vi "Compile Knock Sensor 1.0 Data.vi"(7 "RIO Address":string, 8 "error in (no error)":errorcluster, 11 "Device Item Ref in":T3 format="%.0x") -> (0 "error out":errorcluster, 2 "Knock Sensors":T1[](array[typedef]), 3 "Device Item Ref out":T3 format="%.0x")   [LabVIEW 2020, in "Engine Simulation Toolkit System Explorer.lvlib"]
uses:
  Engine Simulation Toolkit System Explorer.lvlib
  <vilib>/NI VeriStand/Custom Device API/Custom Device Item Ref.ctl
  Shared/1.0 Knock Sensor Engine Data.ctl
  Shared/1.0 Knock Sensor FIFO Idxs.ctl
  Knock Low Freq Setting.ctl
  Shared/Constants and GUIDs.vi
  <vilib>/NI VeriStand/Custom Device Tools/Custom Device Utility Library/NI VeriStand - Search for Item by GUID.vi
  Shared/Properties.vi
  <vilib>/NI VeriStand/Custom Device API/Get Item Property (String).vi
  <vilib>/NI VeriStand/Custom Device API/Get Item Property (U16).vi
  <vilib>/NI VeriStand/Custom Device API/Get Item Property (Double).vi
  Shared/Engine Simulation Toolkit Shared.lvlib
  <vilib>/NI VeriStand/Custom Device Tools/Custom Device Utility Library/Custom Device Utility Library.lvlib
  <vilib>/NI VeriStand/Custom Device API/Custom Device API.lvlib
  <vilib>/rvi/Analysis/host/Public/NI_FpgaMspHost.lvlib
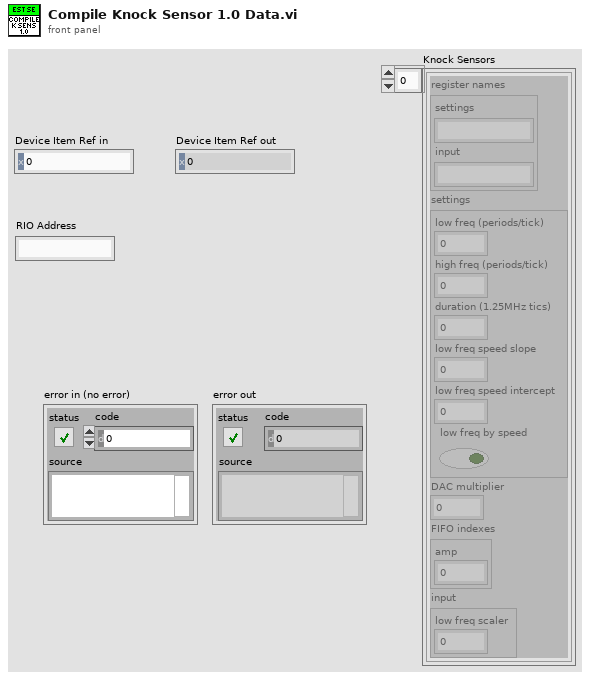
[diagram p1: front panel]
types:
  T1 = typedef "Engine Simulation Toolkit Shared.lvlib/1.0 Knock Sensor Engine Data.ctl" = cluster{"register names":cluster{"settings":string, "input":string}, "settings":cluster{"low freq (periods/tick)":fxp<+,32,0>, "high freq (periods/tick)":fxp<+,32,0>, "duration (1.25MHz tics)":fxp<+,18,18>, "low freq speed slope":fxp<+,16,-3>, "low freq speed intercept":fxp<+,10,-10>, "low freq by speed":bool}, "DAC multiplier":dbl, "FIFO indexes":T2, "input":cluster{"low freq scaler":fxp<+,10,0>}}
  T2 = typedef "Engine Simulation Toolkit Shared.lvlib/1.0 Knock Sensor FIFO Idxs.ctl" = cluster{"amp":i32}
  T3 = typedef "Custom Device API.lvlib/Custom Device Item Ref.ctl" = u64
  T4 = typedef "Engine Simulation Toolkit Shared.lvlib/Channel.ctl" = cluster{"Name":string, "Units":string, "Default":dbl, "Description":string, "Scalable":bool}
  T5 = typedef "Engine Simulation Toolkit System Explorer.lvlib/Knock Low Freq Setting.ctl" = enum16{"Manually", "As function of speed"}
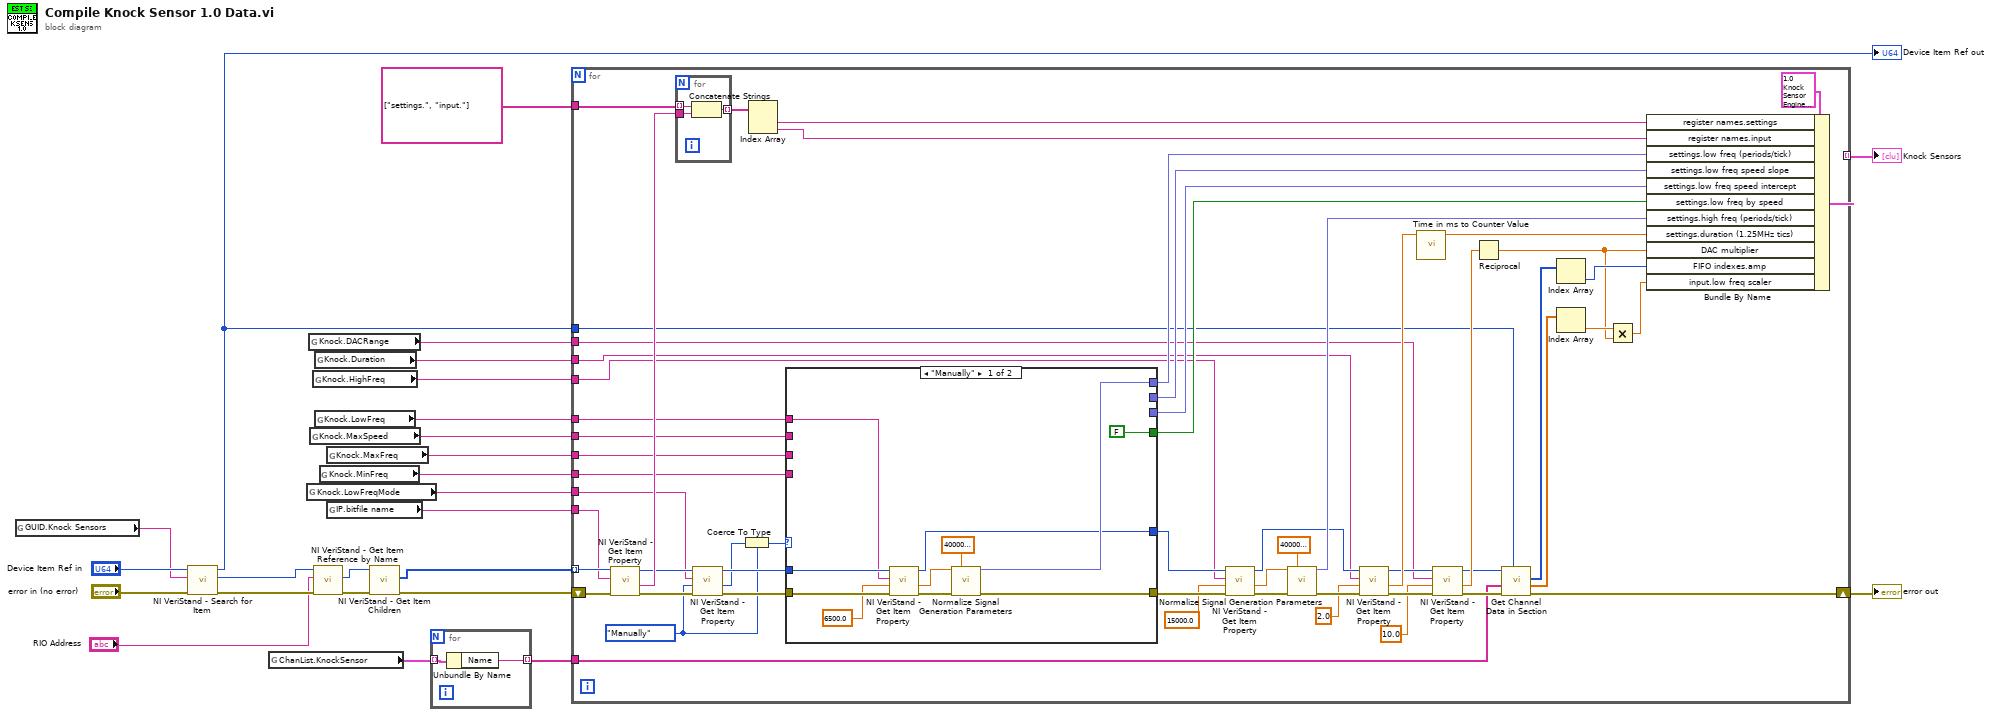
[diagram p0: block diagram]
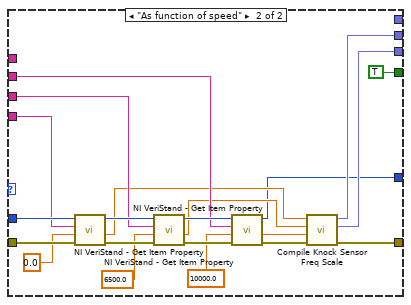
[diagram p2: hidden frame]
diagram:
  n1 = global read "Constants and GUIDs.vi" "GUID.Knock Sensors"() -> (w20:string)
  n2 = call-poly <vilib>:"NI VeriStand - Search for Item.vi"("error in"="error in (no error)", "Item GUID"=w20, "Section Ref in"="Device Item Ref in") -> ("error out"=w5:errorcluster, "Item Ref"=w3:T3, "Section Ref out"=w8:T3)  [unwired: 5 in, 1 out]
  "Device Item Ref out" <- w8
  n3 = global read "Constants and GUIDs.vi" "ChanList.KnockSensor"() -> (w14:T4[])
  n4 = global read "Properties.vi" "Knock.LowFreqMode"() -> (w18:string)
  n5 = global read "Properties.vi" "Knock.DACRange"() -> (w10:string)
  n6 = global read "Properties.vi" "Knock.MaxSpeed"() -> (w15:string)
  n7 = global read "Properties.vi" "Knock.HighFreq"() -> (w9:string)
  n8 = call <vilib>:"NI VeriStand - Get Item Reference by Name.vi"("error in (no error)"=w5, "Item Name"="RIO Address", "Parent Ref in"=w3) -> ("error out"=w6:errorcluster, "Item Ref"=w7:T3)  [unwired: 5 in, 2 out]
  n9 = global read "Properties.vi" "Knock.Duration"() -> (w11:string)
  n10 = global read "Properties.vi" "Knock.LowFreq"() -> (w12:string)
  n11 = global read "Properties.vi" "Knock.MinFreq"() -> (w17:string)
  n12 = global read "Properties.vi" "Knock.MaxFreq"() -> (w16:string)
  n13 = global read "Properties.vi" "IP.bitfile name"() -> (w19:string)
  n14 = call <vilib>:"NI VeriStand - Get Item Children.vi"("error in (no error)"=w6, "Item Ref in"=w7) -> ("error out"=w4:errorcluster, "Child Refs"=w2:T3[])  [unwired: 6 in, 2 out]
  n15 = for {
    tunnel: w14 -> [w27] mode=indexing
    tunnel: [w26] -> w13 mode=indexing
    n16 = Unbundle By Name(w27) -> ("Name"=w26:string)
  }
  n17 = for {
    shift-right: [w38] -> w22
    shift-left: w4 -> [w79]
    tunnel: string[] ["settings.", "input."] -> [w83]
    tunnel: [w81] -> w21 mode=indexing
    tunnel: w2 -> [w78] mode=indexing
    tunnel: w19 -> [w77]
    tunnel: w18 -> [w70]
    tunnel: w17 -> [w69]
    tunnel: w16 -> [w68]
    tunnel: w15 -> [w67]
    tunnel: w13 -> [w35]
    tunnel: w12 -> [w62]
    tunnel: w11 -> [w47]
    tunnel: w10 -> [w41]
    tunnel: w8 -> [w37]
    tunnel: w9 -> [w28]
    w64 = Knock_Low_Freq_Setting."Manually" ("Low frequency (Hz)")
    n18 = call-poly <vilib>:"NI VeriStand - Get Item Property.vi"("error in (no error)"=w79, "Property Name"=w77, "Item Ref in"=w78) -> ("error out"=w72:errorcluster, "Value"=w76:string, "Item Ref out"=w71:T3)  [unwired: 5 in, 1 out]
    n19 = for {
      tunnel: w83 -> [w118] mode=indexing
      tunnel: [w117] -> w80 mode=indexing
      tunnel: w76 -> [w116]
      n20 = Concatenate Strings(w118, w116) -> (w117:string)
    }
    n21 = call-poly <vilib>:"NI VeriStand - Get Item Property.vi"("error in (no error)"=w72, "Default Value"=w64, "Property Name"=w70, "Item Ref in"=w71) -> ("error out"=w73:errorcluster, "Value"=w65:u16, "Item Ref out"=w74:T3)  [unwired: 4 in, 1 out]
    n22 = Coerce To Type(0:w65, 1:w64) -> (2:w63:T5)
    n23 = Index Array(array=w80) -> (element #1=w75:string, element #2=w66:string)  [unwired: 2 in]
    n24 = case shown="\"Manually\"" w63 {
      tunnel: w74 -> [w92 w113]
      tunnel: w73 -> [w94 w112]
      tunnel: w69 -> [_ w109]
      tunnel: w68 -> [_ w108]
      tunnel: w67 -> [_ w107]
      tunnel: [w89 w105] -> w54
      tunnel: [_ w98] -> w59
      tunnel: [_ w97] -> w58
      tunnel: w62 -> [w91 _]
      tunnel: [w86 _] -> w61
      tunnel: [FALSE ("settings.low freq by speed") TRUE ("settings.low freq by speed")] -> w60
      tunnel: [w84 w95] -> w53
      frame "Manually" {
        n25 = call-poly <vilib>:"NI VeriStand - Get Item Property.vi"("error in (no error)"=w94, "Default Value"=6500.0, "Property Name"=w91, "Item Ref in"=w92) -> ("error out"=w93:errorcluster, "Value"=w88:dbl, "Item Ref out"=w84:T3)  [unwired: 4 in, 1 out]
        n26 = call <vilib>:"Normalize Signal Generation Parameters.vi"("frequency (Hz)"=w88, "FPGA clock rate (Hz)"=40000000.0, "error in (no error)"=w93) -> ("frequency (periods/tick)"=w86:fxp<+,32,0>, "error out"=w89:errorcluster)  [unwired: 7 in, 4 out]
      }
      frame "As function of speed" {
        n27 = call-poly <vilib>:"NI VeriStand - Get Item Property.vi"("error in (no error)"=w112, "Default Value"=0.0, "Property Name"=w109, "Item Ref in"=w113) -> ("error out"=w110:errorcluster, "Value"=w104:dbl, "Item Ref out"=w111:T3)  [unwired: 4 in, 1 out]
        n28 = call-poly <vilib>:"NI VeriStand - Get Item Property.vi"("error in (no error)"=w110, "Default Value"=6500.0, "Property Name"=w108, "Item Ref in"=w111) -> ("error out"=w115:errorcluster, "Value"=w100:dbl, "Item Ref out"=w114:T3)  [unwired: 4 in, 1 out]
        n29 = call-poly <vilib>:"NI VeriStand - Get Item Property.vi"("error in (no error)"=w115, "Default Value"=10000.0, "Property Name"=w107, "Item Ref in"=w114) -> ("error out"=w106:errorcluster, "Value"=w99:dbl, "Item Ref out"=w95:T3)  [unwired: 4 in, 1 out]
        n30 = call "Compile Knock Sensor Freq Scale.vi"("error in (no error)"=w106, "max rpm"=w99, "max freq"=w100, "min freq"=w104) -> ("error out"=w105:errorcluster, "fxp intercept (b)"=w97:fxp<+,10,-10>, "fxp slope (m)"=w98:fxp<+,16,-3>)  [unwired: 5 in]
      }
    }
    n31 = call-poly <vilib>:"NI VeriStand - Get Item Property.vi"("error in (no error)"=w54, "Default Value"=15000.0, "Property Name"=w28, "Item Ref in"=w53) -> ("error out"=w55:errorcluster, "Value"=w56:dbl, "Item Ref out"=w48:T3)  [unwired: 4 in, 1 out]
    n32 = call <vilib>:"Normalize Signal Generation Parameters.vi"("frequency (Hz)"=w56, "FPGA clock rate (Hz)"=40000000.0, "error in (no error)"=w55) -> ("frequency (periods/tick)"=w50:fxp<+,32,0>, "error out"=w51:errorcluster)  [unwired: 7 in, 4 out]
    n33 = call-poly <vilib>:"NI VeriStand - Get Item Property.vi"("error in (no error)"=w51, "Default Value"=2.0, "Property Name"=w47, "Item Ref in"=w48) -> ("error out"=w49:errorcluster, "Value"=w45:dbl, "Item Ref out"=w42:T3)  [unwired: 4 in, 1 out]
    n34 = call "Time in ms to Counter Value.vi"("time (ms)"=w45) -> ("counter value"=w44:dbl)  [unwired: 10 in]
    n35 = call-poly <vilib>:"NI VeriStand - Get Item Property.vi"("error in (no error)"=w49, "Default Value"=10.0, "Property Name"=w41, "Item Ref in"=w42) -> ("error out"=w43:errorcluster, "Value"=w39:dbl, "Item Ref out"=w36:T3)  [unwired: 4 in, 1 out]
    n36 = Reciprocal(x=w39) -> (1/x=w30:dbl)
    n37 = call "Get Channel Data in Section.vi"("Custom device ref"=w37, "error in (no error)"=w43, "Channels"=w35, "Item Ref in"=w36) -> ("error out"=w38:errorcluster, "default values"=w32:dbl[], "FIFO indexes"=w34:i32[])  [unwired: 3 in, 2 out]
    n38 = Index Array(array=w34) -> (element=w33:i32)  [unwired: 1 in]
    n39 = Index Array(array=w32) -> (element=w31:dbl)  [unwired: 1 in]
    n40 = Multiply(x=w31, y=w30) -> (x*y=w29:dbl)
    n41 = Bundle By Name(cluster=T1 {"register names"={"settings"="", "input"=""}, "settings"={"low freq (periods/tick)"=0.0, "high freq (periods/tick)"=0.0, "duration (1.25MHz tics)"=0.0, "low freq speed slope"=0.0, "low freq speed intercept"=0.0, "low freq by speed"=FALSE}, "DAC multiplier"=0.0, "FIFO indexes"={"amp"=0}, "input"={"low freq scaler"=0.0}} ("1.0.0 Knock Sensor"), "register names.settings"=w75, "register names.input"=w66, "settings.low freq (periods/tick)"=w61, "settings.low freq speed slope"=w59, "settings.low freq speed intercept"=w58, "settings.low freq by speed"=w60, "settings.high freq (periods/tick)"=w50, "settings.duration (1.25MHz tics)"=w44, "DAC multiplier"=w30, "FIFO indexes.amp"=w33, "input.low freq scaler"=w29) -> (w81:T1)
  }
  "error out" <- w22
  "Knock Sensors" <- w21
